vi "TemperatureConverter.vi"() -> ()   [LabVIEW 2019]
panel:
  out "Output":dbl
  in  "Input":dbl
  in  "Enum":T1(ring)
  # "(derajat C) = 9/5 derajat Celsius + 32\n(K) =  derajat C + 273\n(derajat C) = 5/9 derajat F – 32\n(K) = 5/9 ( derajat F – 32) + 273\n(derajat F) = 9/4  derajat F + 32\n(K) = 5/4 T derajat R + 273\n(derajat C) = K – 273\n(derajat F) = 9/5 (T-273) + 32"
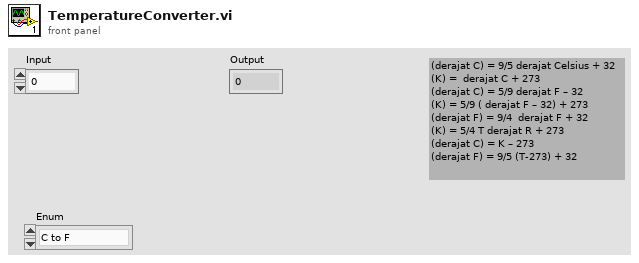
[diagram p1: front panel]
types:
  T1 = enum16{"C to F", "F to C", "K to F", "F to K", "C to K", "K to C"}
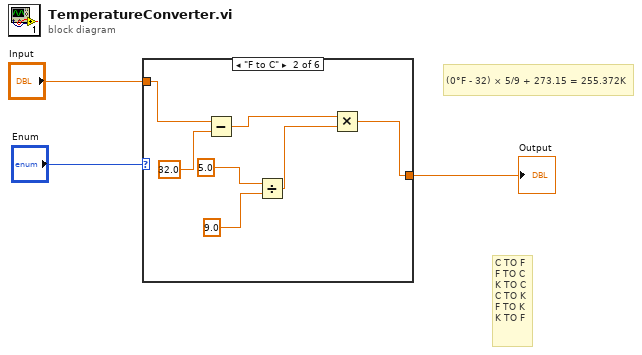
[diagram p0: block diagram]
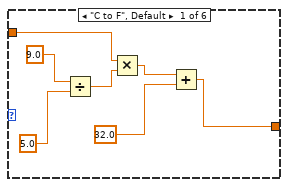
[diagram p2: hidden frame]
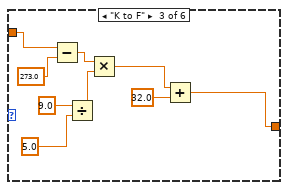
[diagram p3: hidden frame]
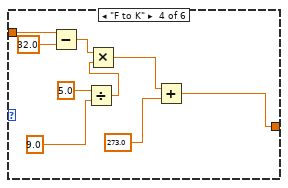
[diagram p4: hidden frame]
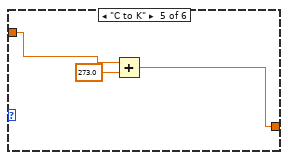
[diagram p5: hidden frame]
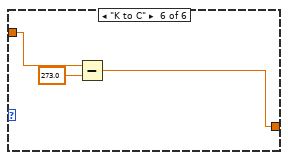
[diagram p6: hidden frame]
diagram:
  # "(0°F - 32) × 5/9 + 273.15 = 255.372K"
  # "C TO F\nF TO C\nK TO C\nC TO K\nF TO K\nK TO F"
  n1 = case shown="\"F to C\"" "Enum" {
    tunnel: "Input" -> [w7 w17 w26 w35 w38 w41]
    tunnel: [w4 w11 w18 w27 w36 w39] -> w1
    frame "C to F", Default {
      n2 = Divide(x=9.0, y=5.0) -> (x/y=w8:dbl)
      n3 = Multiply(x=w7, y=w8) -> (x*y=w6:dbl)
      n4 = Add(x=w6, y=32.0) -> (x+y=w4:dbl)
    }
    frame "F to C" {
      n5 = Subtract(x=w17, y=32.0) -> (x-y=w15:dbl)
      n6 = Divide(x=5.0, y=9.0) -> (x/y=w12:dbl)
      n7 = Multiply(x=w15, y=w12) -> (x*y=w11:dbl)
    }
    frame "K to F" {
      n8 = Subtract(x=w26, y=273.0) -> (x-y=w23:dbl)
      n9 = Divide(x=9.0, y=5.0) -> (x/y=w24:dbl)
      n10 = Multiply(x=w23, y=w24) -> (x*y=w20:dbl)
      n11 = Add(x=w20, y=32.0) -> (x+y=w18:dbl)
    }
    frame "F to K" {
      n12 = Subtract(x=w35, y=32.0) -> (x-y=w30:dbl)
      n13 = Divide(x=5.0, y=9.0) -> (x/y=w31:dbl)
      n14 = Multiply(x=w30, y=w31) -> (x*y=w29:dbl)
      n15 = Add(x=w29, y=273.0) -> (x+y=w27:dbl)
    }
    frame "C to K" {
      n16 = Add(x=w38, y=273.0) -> (x+y=w36:dbl)
    }
    frame "K to C" {
      n17 = Subtract(x=w41, y=273.0) -> (x-y=w39:dbl)
    }
  }
  "Output" <- w1
